vi "Test CPC Comm.vi"() -> ()   [LabVIEW 2012]
uses:
  CPC.lvclass
panel:
  out "error out 2":errorcluster
  out "FP Conc":dbl
  out "error out":errorcluster
  in  "Boolean":bool
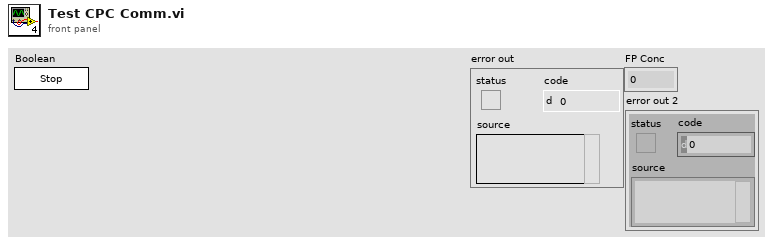
[diagram p1: front panel]
types:
  T1 = cluster{"baud rate (9600)":u32, "data bits (8)":u16, "stop bits (10: 1 bit)":u16, "parity (0:none)":enum16{"None", "Odd", "Even", "Mark", "Space"}, "flow control (0:none)":u16, "endModeforReads":u16, "endModeforWrites":u16}
  T2 = cluster{"EnTermChar":bool, "termChar":u8, "suppEnEnRd":bool, "sendEndEn":bool}
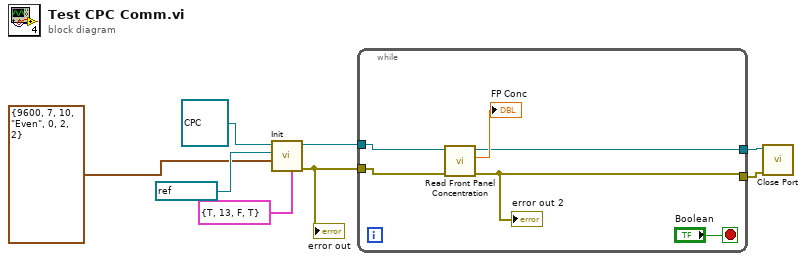
[diagram p0: block diagram]
diagram:
  n1 = call-dynamic "Init.vi"("Message Cfg"=T2 {"EnTermChar"=TRUE, "termChar"=13, "suppEnEnRd"=FALSE, "sendEndEn"=TRUE}, "serialCfg"=T1 {"baud rate (9600)"=9600, "data bits (8)"=7, "stop bits (10: 1 bit)"=10, "parity (0:none)"=enum."Even", "flow control (0:none)"=0, "endModeforReads"=2, "endModeforWrites"=2}, "Port"=refnum<visa-resource-name> "COM4", "CPC in"=refnum<class "CPC.lvclass"> refnum ("CPC.lvclass")) -> ("error out"=w5:errorcluster, "CPC out"=w6:refnum<class "CPC.lvclass">)  [unwired: 6 in]
  "error out" <- w5
  n2 = while {
    tunnel: w6 -> [w13]
    tunnel: w5 -> [w12]
    tunnel: [w10] -> w4
    tunnel: [w9] -> w3
    stop <- "Boolean" stop-if-true
    n3 = call "Read Front Panel Concentration.vi"("error in (no error)"=w12, "CPC in"=w13) -> ("error out"=w10:errorcluster, "FP Conc"=→"FP Conc":dbl, "CPC out"=w9:refnum<class "CPC.lvclass">)  [unwired: 7 in]
    "error out 2" <- w10
  }
  n4 = call-dynamic "Close Port.vi"("error in (no error)"=w4, "Serial IO in"=w3) -> ()  [unwired: 8 in, 2 out]
